vi "ExSubCreateFileDisplayMultImageDPH.vi"(0 "Camera Handle":u32, 1 "Pulser Handle":u32, 2 "file handle":u32, 3 "error in (no error)":errorcluster, 4 "Number of Images":u16=1 min=1 step=1) -> (5 "Handles Out":T1, 6 "Array":u32[](array[numeric]), 7 "error out":errorcluster)   [LabVIEW 2015]
panel:
  # "ExSubCreateFileDisplayMultImage.vi:\nThis is a SubVI that creates a file, display and image objects and returns the handles bundled in a cluster that includes a pulser and camera handle"
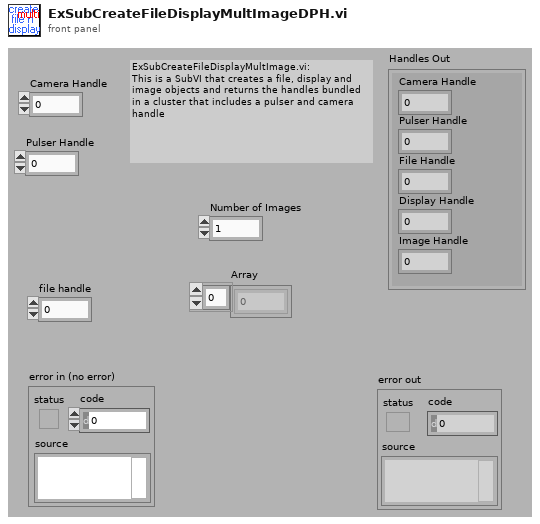
[diagram p1: front panel]
types:
  T1 = cluster{"Camera Handle":u32, "Pulser Handle":u32, "File Handle":u32, "Display Handle":u32, "Image Handle":u32}
  T2 = cluster{"Camera Handle":u32, "Pulser Handle":u32, "file handle":u32, i32, "Image Handle":u32}
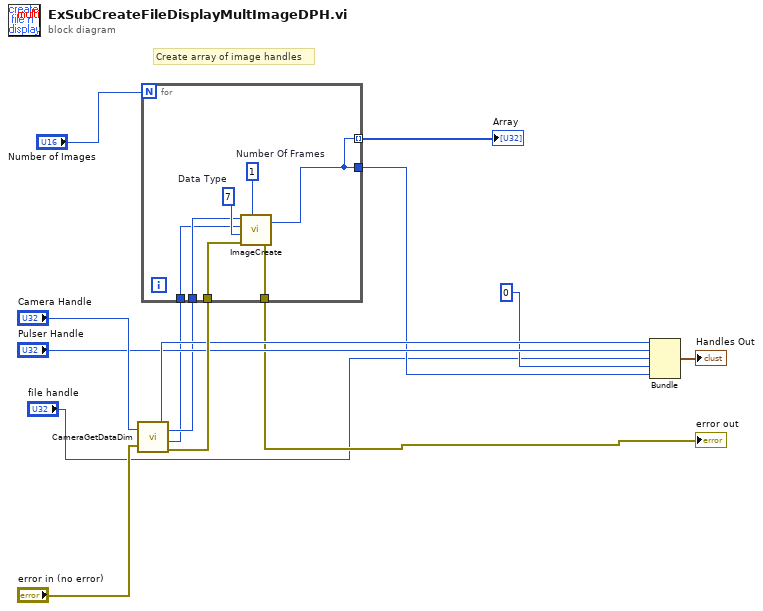
[diagram p0: block diagram]
diagram:
  # "Create array of image handles"
  n1 = call <userlib>:"CameraGetDataDim.vi"("Camera Handle"="Camera Handle", "error in"="error in (no error)") -> ("Camera Handle"=w11:u32, "Xdim"=w6:u32, "Ydim"=w5:u32, "error out"=w14:errorcluster)
  n2 = for {
    N: "Number of Images" -> [_]
    tunnel: w14 -> [w21]
    tunnel: [w20] -> w3
    tunnel: [w15] -> w9
    tunnel: w6 -> [w17]
    tunnel: w5 -> [w16]
    tunnel: [w15] -> w1 mode=indexing
    w18 = u32 1  # Number Of Frames
    w19 = u32 7  # Data Type
    n3 = call <userlib>:"ImageCreate.vi"("X dimension"=w17, "Y dimension"=w16, "Data Type"=w19, "error in"=w21, "Number Of Frames"=w18) -> ("Image Handle"=w15:u32, "error out"=w20:errorcluster)
  }
  "error out" <- w3
  "Array" <- w1
  n4 = Bundle("Camera Handle"=w11, "Pulser Handle"="Pulser Handle", "file handle"="file handle", 0, "Image Handle"=w9) -> (→"Handles Out":T2)  [unwired: 1 in]
